vi "Read Columns.vi"(8 "error in (no error)":errorcluster, 11 "Line in":refnum<class "Line.lvclass">) -> (0 "error out":errorcluster, 2 "Columns":refnum<class "Column.lvclass">[](array[class]), 3 "Line out":refnum<class "Line.lvclass">)   [LabVIEW 2013, in "Table Manager.lvlib" / "Line.lvclass"]
uses:
  Line.lvclass
  Column/Column.lvclass
  Line.lvclass/Line.ctl
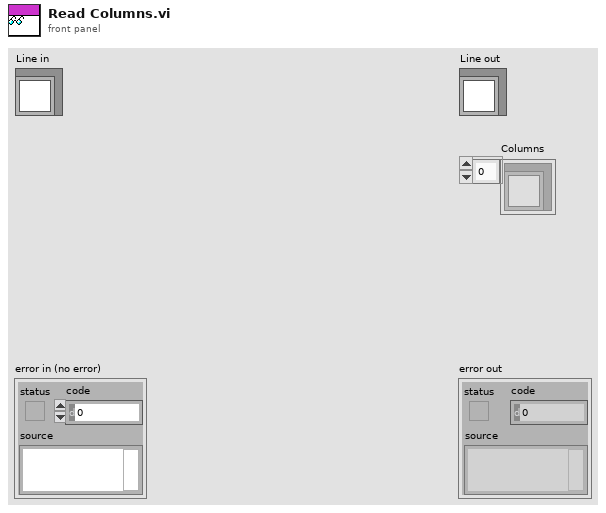
[diagram p1: front panel]
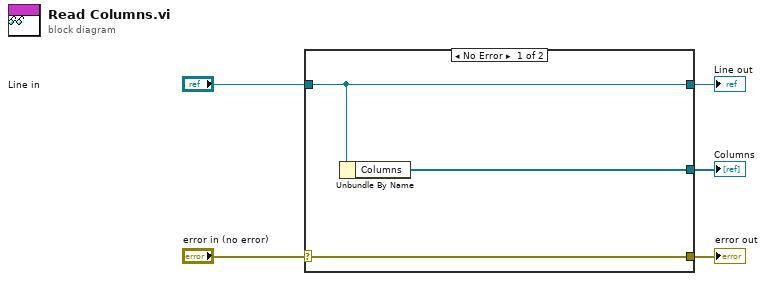
[diagram p0: block diagram]
diagram:
  n1 = case shown="No Error" "error in (no error)" {
    selector: "error in (no error)" -> [w8 w9]
    tunnel: [w8 w9] -> w4
    tunnel: [w7 w10] -> w2
    tunnel: "Line in" -> [w7 w10]
    tunnel: [w6 _] -> w1
    frame No Error {
      n2 = Unbundle By Name(w7) -> ("Columns"=w6:refnum<class "Column.lvclass">[])
    }
    frame Error {
    }
  }
  "error out" <- w4
  "Line out" <- w2
  "Columns" <- w1
